vi "initialize_data_log.vi"(7 "Overwrite?":bool, 8 "error in (no error)":errorcluster, 9 "Initialization Data":variant, 10 "Path":path, 11 "data_logger in":refnum<class "data_logger.lvclass">) -> (0 "error out":errorcluster, 3 "data_logger out":refnum<class "data_logger.lvclass">)   [LabVIEW 2015, in "data_logger.lvclass"]
uses:
  data_logger.lvclass
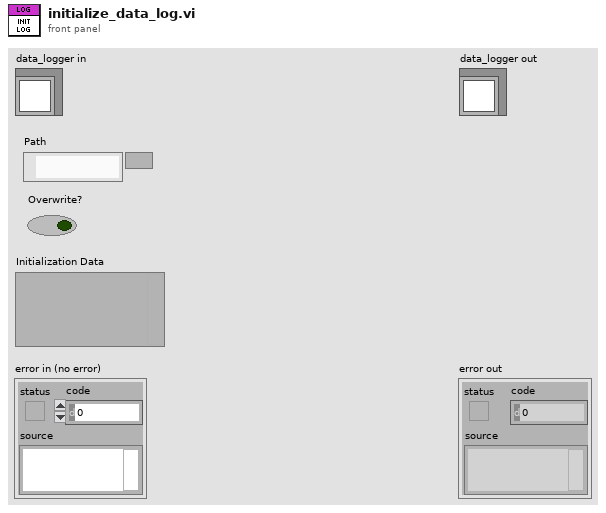
[diagram p1: front panel]
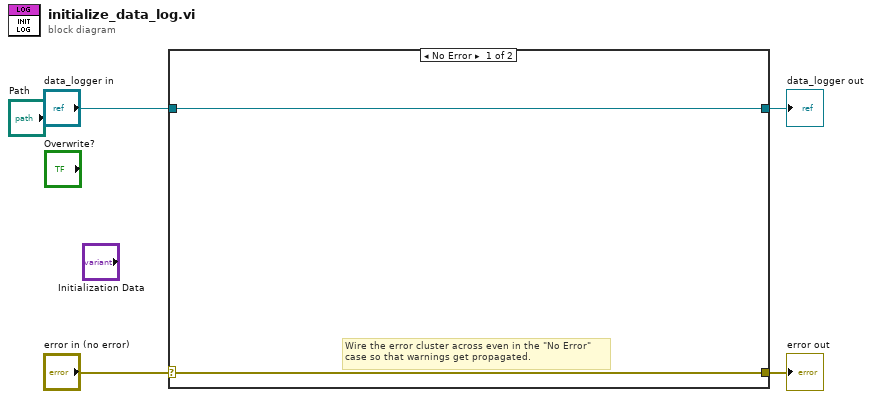
[diagram p0: block diagram]
diagram:
  n1 = case shown="No Error" "error in (no error)" {
    selector: "error in (no error)" -> [w5 w8]
    tunnel: [w5 w8] -> w3
    tunnel: [w6 w7] -> w1
    tunnel: "data_logger in" -> [w6 w7]
    frame No Error {
      # "Wire the error cluster across even in the \"No Error\"\ncase so that warnings get propagated."
    }
    frame Error {
    }
  }
  "error out" <- w3
  "data_logger out" <- w1
